vi "Acquire Image.vi"(7 "Camera ID":u8, 8 "error in (no error)":errorcluster, 10 "EXE path":path, 11 "Save to":path=path "C:/batt/test.jpg") -> (0 "error out":errorcluster, 3 "Image path":path)   [LabVIEW 2025]
doc: "Uses an external app to acquire a JPEG image from a webcam."
panel:
  out "2D Picture":picture
  out "standard error":string
  out "return code":i32
  out "standard output":string
  out "args":string
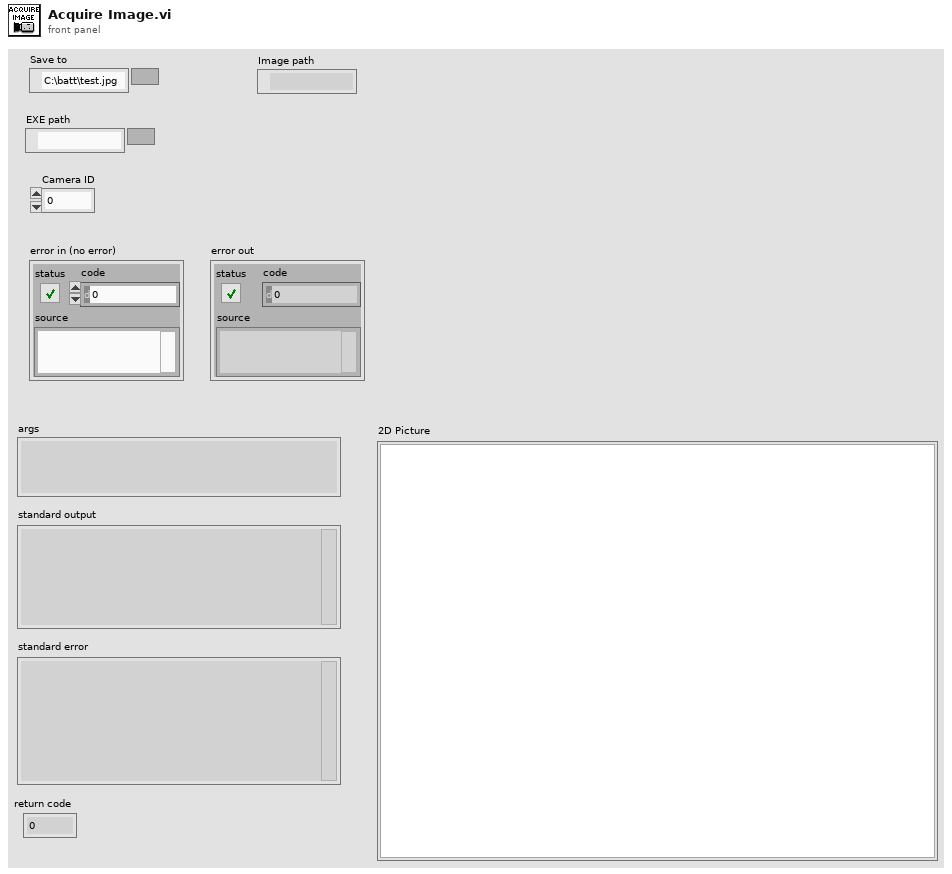
[diagram p1: front panel]
types:
  T1 = typedef "imagedata.ctl" = cluster{"image type":i32, "image depth":i32, "image":u8[], "mask":u8[], "colors":u32[], "Rectangle":cluster{"left":i16, "top":i16, "right":i16, "bottom":i16}}
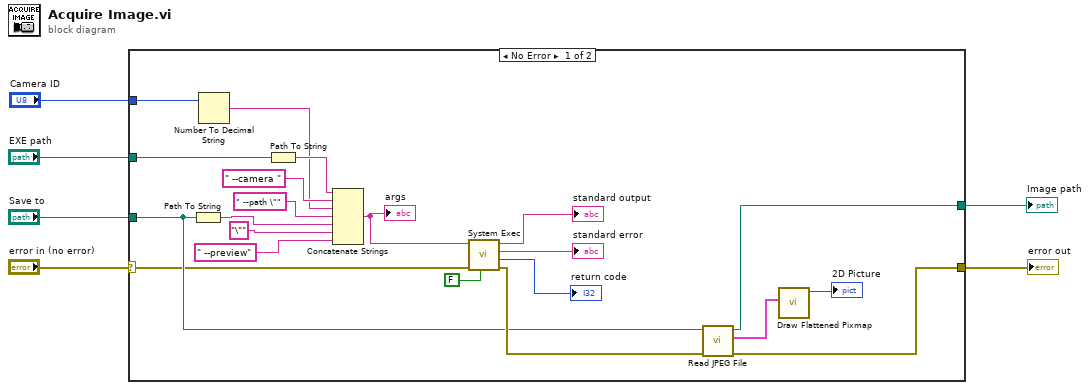
[diagram p0: block diagram]
diagram:
  n1 = case shown="No Error" "error in (no error)" {
    selector: "error in (no error)" -> [w11 w28]
    tunnel: "EXE path" -> [w13 _]
    tunnel: "Save to" -> [w12 _]
    tunnel: [w10 w28] -> w3
    tunnel: [w9 _] -> w2
    tunnel: "Camera ID" -> [w8 _]
    frame No Error {
      n2 = Path To String(path=w12) -> (string=w17:string)
      n3 = Number To Decimal String(number=w8) -> (decimal integer string=w7:string)  [unwired: 1 in]
      n4 = Path To String(path=w13) -> (string=w19:string)
      n5 = Concatenate Strings(w19, " --camera " ("string"), w7, " --path \"", w17, "\"" ("string"), " --preview" ("string")) -> (w24:string)
      "args" <- w24
      n6 = call <vilib>:"System Exec.vi"("run minimized? (F)"=FALSE, "error in (no error)"=w11, "command line"=w24) -> ("error out"=w16:errorcluster, "return code"=→"return code":i32, "standard error"=→"standard error":string, "standard output"=→"standard output":string)  [unwired: 5 in]
      n7 = call <vilib>:"Read JPEG File.vi"("error in (no error)"=w16, "path to JPEG file"=w12) -> ("error out"=w10:errorcluster, "image data"=w15:T1, "path"=w9:path)  [unwired: 7 in]
      n8 = call <vilib>:"Draw Flattened Pixmap.vi"("image data"=w15) -> ("new picture"=→"2D Picture":picture)  [unwired: 8 in]
    }
    frame Error {
    }
  }
  "error out" <- w3
  "Image path" <- w2
